vi "Quiz #1.vi"() -> ()   [LabVIEW 2019]
panel:
  out "String":string
  out "x+y":dbl
  out "subarray":dbl[](array[numeric])
  out "ANGULOS":dbl[](array[numeric])
  in  "COORDENADA Y":dbl format="%#_26g"
  in  "COORDENADA X":dbl format="%#_21g"
  out "VECTORES B":dbl[](array[numeric])
  out "VECTORES A":dbl[](array[numeric])
  in  "Y":dbl[](array[numeric]) format="%#_21g"
  in  "X":dbl[](array[numeric]) format="%#_21g"
  out "PUNTOS COORDENADOS":cluster{"X":dbl[], "Y":dbl[]}(graph)
  out "B2":dbl
  out "B1":dbl
  out "A2":dbl
  out "A1":dbl
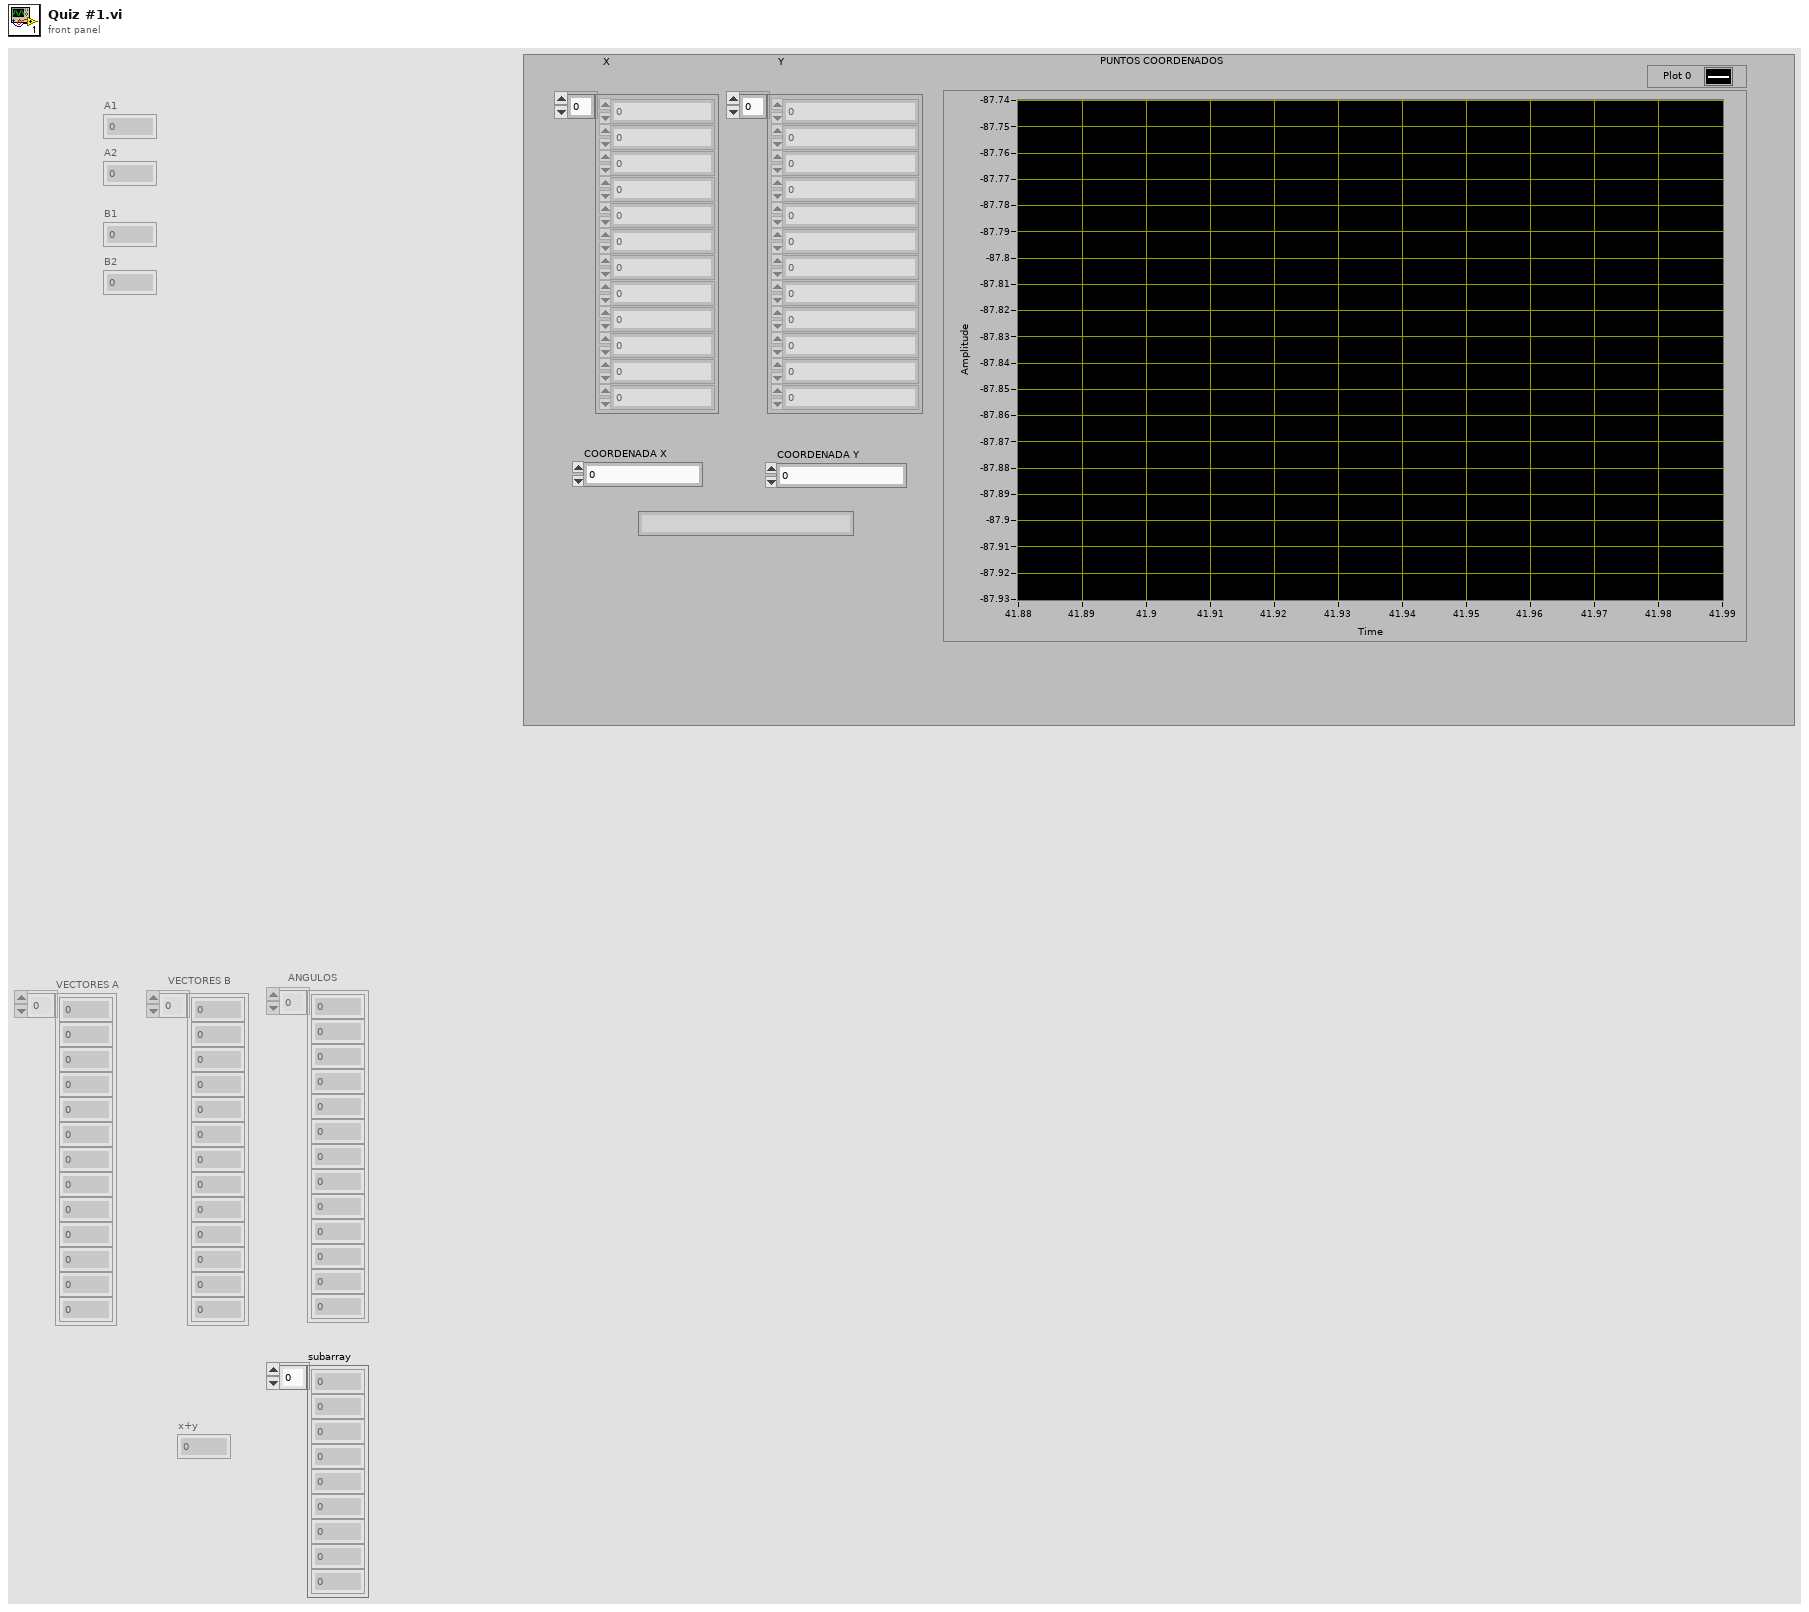
[diagram p1: front panel]
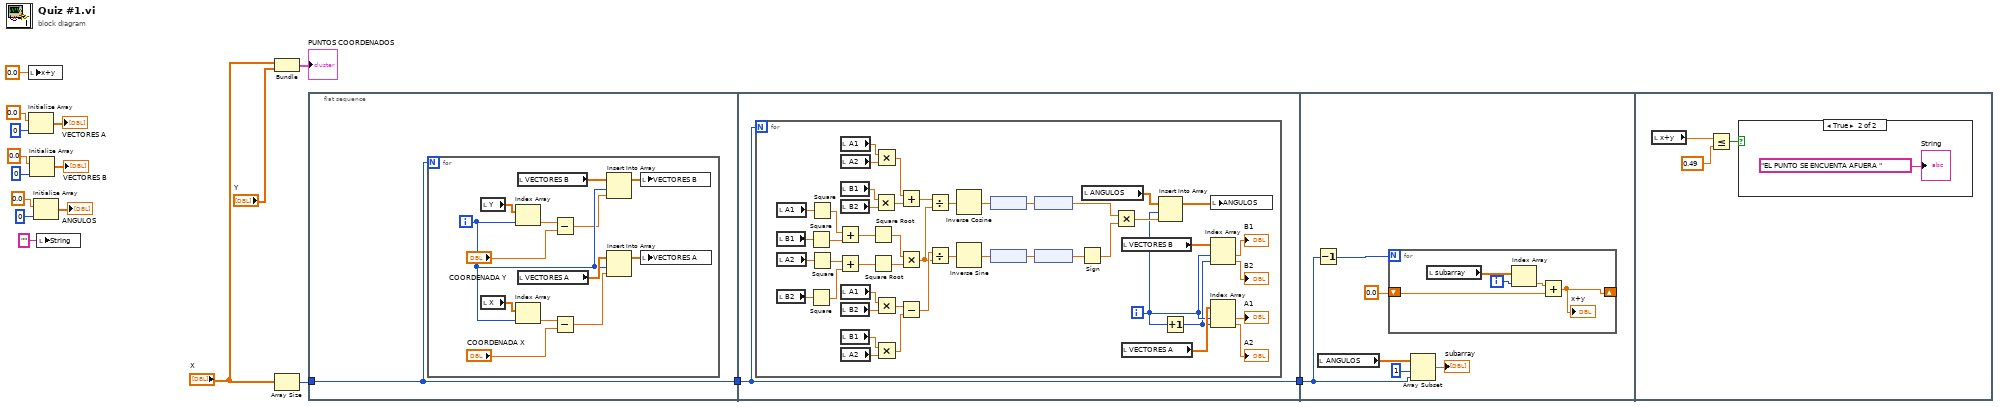
[diagram p0: block diagram]
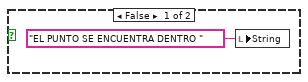
[diagram p2: hidden frame]
diagram:
  n1 = local write "x+y"(0.0 ("x+y")) -> ()
  n2 = Initialize Array(0.0 ("element"), 0 ("dimension size")) -> (→"VECTORES A":dbl[])
  n3 = Initialize Array(0.0 ("element"), 0 ("dimension size")) -> (→"VECTORES B":dbl[])
  n4 = Initialize Array(0.0 ("element"), 0 ("dimension size")) -> (→"ANGULOS":dbl[])
  n5 = local write "String"("" ("String")) -> ()
  n6 = Bundle("X"="X", "Y"="Y") -> (→"PUNTOS COORDENADOS":cluster{"X":dbl[], "Y":dbl[]})  [unwired: 1 in]
  n7 = Array Size(array="X") -> (size(s)=w5:i32)
  n8 = flat-sequence {
    tunnel: w5 -> [w18]
    tunnel: [w18] -> w4
    tunnel: w4 -> [w32]
    tunnel: [w32] -> w3
    tunnel: w3 -> [w81]
    frame #0 {
      n9 = for {
        N: w18 -> [_]
        i -> [w22]
        n10 = local read "Y"() -> (w31:dbl[])
        n11 = local read "X"() -> (w30:dbl[])
        n12 = Index Array(array=w31, index=w22) -> (element=w27:dbl)
        n13 = Index Array(array=w30, index=w22) -> (element=w29:dbl)
        n14 = local read "VECTORES B"() -> (w19:dbl[])
        n15 = local read "VECTORES A"() -> (w23:dbl[])
        n16 = Subtract(x=w27, y="COORDENADA Y") -> (x-y=w21:dbl)
        n17 = Subtract(x=w29, y="COORDENADA X") -> (x-y=w25:dbl)
        n18 = Insert Into Array(array=w19, index=w22, new element=w21) -> (w20:dbl[])
        n19 = Insert Into Array(array=w23, index=w22, new element=w25) -> (w24:dbl[])
        n20 = local write "VECTORES B"(w20) -> ()
        n21 = local write "VECTORES A"(w24) -> ()
      }
    }
    frame #1 {
      n22 = for {
        N: w32 -> [_]
        i -> [w48]
        n23 = local read "A1"() -> (w79:dbl)
        n24 = local read "B1"() -> (w77:dbl)
        n25 = local read "A2"() -> (w75:dbl)
        n26 = local read "B2"() -> (w74:dbl)
        n27 = Square(x=w77) -> (x^2=w78:dbl)
        n28 = Square(x=w74) -> (x^2=w73:dbl)
        n29 = Square(x=w79) -> (x^2=w76:dbl)
        n30 = Square(x=w75) -> (x^2=w72:dbl)
        n31 = Add(x=w76, y=w78) -> (x+y=w71:dbl)
        n32 = Add(x=w72, y=w73) -> (x+y=w68:dbl)
        n33 = local read "A1"() -> (w39:dbl)
        n34 = local read "A2"() -> (w40:dbl)
        n35 = local read "B1"() -> (w41:dbl)
        n36 = local read "B2"() -> (w42:dbl)
        n37 = local read "A1"() -> (w67:dbl)
        n38 = local read "B2"() -> (w66:dbl)
        n39 = local read "B1"() -> (w65:dbl)
        n40 = local read "A2"() -> (w64:dbl)
        n41 = Square Root(x=w71) -> (sqrt(x)=w70:dbl)
        n42 = Square Root(x=w68) -> (sqrt(x)=w69:dbl)
        n43 = Multiply(x=w41, y=w42) -> (x*y=w37:dbl)
        n44 = Multiply(x=w39, y=w40) -> (x*y=w38:dbl)
        n45 = Multiply(x=w67, y=w66) -> (x*y=w63:dbl)
        n46 = Multiply(x=w65, y=w64) -> (x*y=w62:dbl)
        n47 = Add(x=w38, y=w37) -> (x+y=w36:dbl)
        n48 = Multiply(x=w70, y=w69) -> (x*y=w35:dbl)
        n49 = Subtract(x=w63, y=w62) -> (x-y=w61:dbl)
        n50 = Divide(x=w36, y=w35) -> (x/y=w54:dbl)
        n51 = Divide(x=w61, y=w35) -> (x/y=w34:dbl)
        n52 = Inverse Cosine(1:w54) -> (0:w51:dbl)
        n53 = Inverse Sine(1:w34) -> (0:w33:dbl)
        n54 = node(w51) -> (w52:dbl[unit])
        n55 = node(w33) -> (w60:dbl[unit])
        n56 = node(w52) -> (w53:dbl)
        n57 = node(w60) -> (w59:dbl)
        n58 = Sign(1:w59) -> (0:w58:dbl)
        n59 = local read "ANGULOS"() -> (w55:dbl[])
        n60 = Multiply(x=w53, y=w58) -> (x*y=w57:dbl)
        n61 = local read "VECTORES B"() -> (w49:dbl[])
        n62 = local read "VECTORES A"() -> (w50:dbl[])
        n63 = Insert Into Array(array=w55, index=w48, new element=w57) -> (w56:dbl[])
        n64 = Increment(x=w48) -> (x+1=w47:i32)
        n65 = local write "ANGULOS"(w56) -> ()
        n66 = Index Array(array=w49, index #1=w48, index #2=w47) -> (element #1=→"B1":dbl, element #2=→"B2":dbl)
        n67 = Index Array(array=w50, index #1=w48, index #2=w47) -> (element #1=→"A1":dbl, element #2=→"A2":dbl)
      }
    }
    frame #2 {
      n68 = Decrement(x=w81) -> (x-1=w82:i32)
      n69 = local read "ANGULOS"() -> (w85:dbl[])
      n70 = for {
        N: w82 -> [_]
        shift-right: [w87] -> _
        shift-left: 0.0 -> [w86]
        i -> [w89]
        n71 = local read "subarray"() -> (w90:dbl[])
        n72 = Index Array(array=w90, index=w89) -> (element=w88:dbl)
        n73 = Add(x=w88, y=w86) -> (x+y=w87:dbl)
        "x+y" <- w87
      }
      n74 = Array Subset(array=w85, index=1, length=w81) -> (→"subarray":dbl[])
    }
    frame #3 {
      n75 = local read "x+y"() -> (w93:dbl)
      n76 = Less Or Equal?(x=w93, y=0.49) -> (x <= y?=w91:bool)
      n77 = case shown="True" w91 {
        frame False {
          n78 = local write "String"("EL PUNTO SE ENCUENTRA DENTRO " ("String")) -> ()
        }
        frame True {
          "String" <- "EL PUNTO SE ENCUENTA AFUERA "
        }
      }
    }
  }
